vi "Convert Complex Data To Waveform.vi"(8 "error in":errorcluster, 9 "Real Data":fxp<+/-,21,14>[](array[numeric]), 10 "Imaginary Data":fxp<+/-,21,14>[](array[numeric]), 11 "Sample Rate (S/s)":dbl) -> (0 "error out":errorcluster, 3 "Waveform":waveform(dbl))   [LabVIEW 2014]
doc: "This VI turns an array of 256 complex signal data points into Waveform data for easy display on a chart or graph."
uses:
  <vilib>/rvi/Analysis/host/Public/NI_FpgaMspHost.lvlib
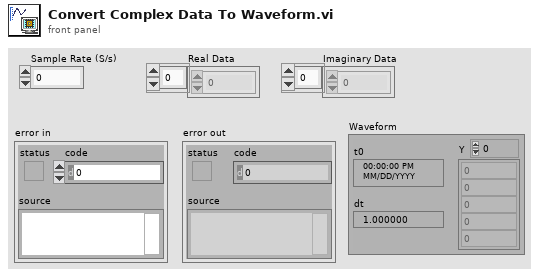
[diagram p1: front panel]
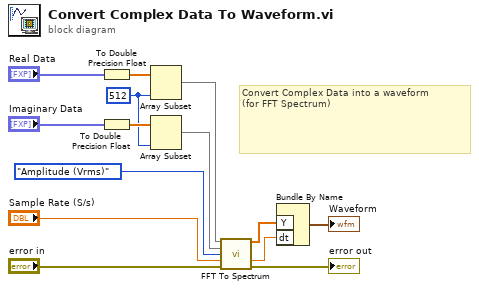
[diagram p0: block diagram]
diagram:
  w5 = 512 ("length")
  # "Convert Complex Data into a waveform\n(for FFT Spectrum)"
  n1 = To Double Precision Float(number="Real Data") -> (double precision float=w4:dbl[])
  n2 = To Double Precision Float(number="Imaginary Data") -> (double precision float=w6:dbl[])
  n3 = Array Subset(array=w4, length=w5) -> (w8:dbl[])  [unwired: 1 in]
  n4 = Array Subset(array=w6, length=w5) -> (w9:dbl[])  [unwired: 1 in]
  n5 = call <vilib>:"FFT To Spectrum.vi"("real FFT data"=w8, "imaginary FFT data"=w9, "spectrum type"=enum8{"Power (Vrms^2)", "Amplitude (Vrms)"}."Amplitude (Vrms)", "sample rate (S/s)"="Sample Rate (S/s)", "error in (no error)"="error in") -> ("spectrum out"=w12:dbl[], "df (Hz)"=w13:dbl, "error out"=→"error out":errorcluster)  [unwired: 8 in]
  n6 = Bundle By Name("Y"=w12, "dt"=w13) -> (→"Waveform":waveform(dbl))  [unwired: 1 in]
